vi "List Unacknowledged Packets.vi"(8 "error in (no error)":errorcluster, 9 "filter (0s: list all)":dbl, 11 "Subscription in":refnum<class "Subscription.lvclass">) -> (0 "error out":errorcluster, 2 "Unacknowledged":T1[](array[typedef]), 3 "Subscription out":refnum<class "Subscription.lvclass">)   [LabVIEW 2013, in "MQTT Server.lvlib" / "Subscription.lvclass"]
uses:
  Subscription.lvclass
  Stored Packet -- cluster.ctl
  <vilib>/LabVIEW Open Source Project/MQTT Control Packets/Control Packets/ControlPacket/ControlPacket.lvclass
  Subscription.lvclass/Subscription.ctl
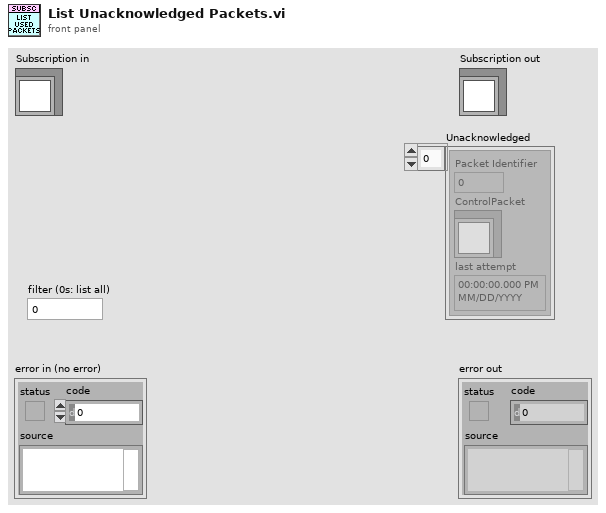
[diagram p1: front panel]
types:
  T1 = typedef "MQTT Server.lvlib/Subscription.lvclass/Stored Packet -- cluster.ctl" = cluster{"Packet Identifier":u16, "ControlPacket":refnum<class "ControlPacket.lvclass">, "last attempt":timestamp}
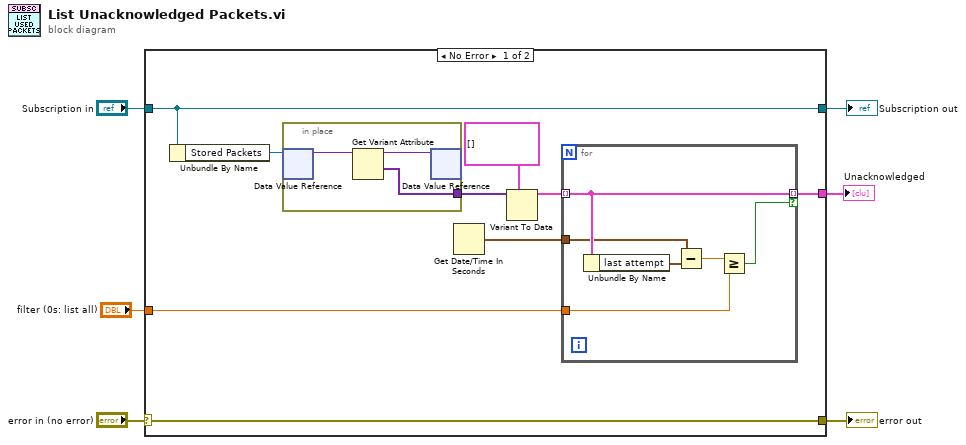
[diagram p0: block diagram]
diagram:
  n1 = case shown="No Error" "error in (no error)" {
    selector: "error in (no error)" -> [w15 w26]
    tunnel: [w15 w26] -> w5
    tunnel: [w14 w25] -> w3
    tunnel: "Subscription in" -> [w14 w25]
    tunnel: [w9 _] -> w2
    tunnel: "filter (0s: list all)" -> [w8 _]
    frame No Error {
      n2 = Unbundle By Name(w14) -> ("Stored Packets"=w13:refnum<data-value>)
      n3 = in-place {
        in-place-border: [w22] -> w12
        n4 = in-place-dvr #1(w13) -> (w24:variant)  [unwired: 1 out]
        n5 = Get Variant Attribute(Variant=w24) -> (duplicate Variant=w23:variant, values=w22:variant[])  [unwired: 3 in, 2 out]
        n6 = in-place-dvr #1(w23) -> ()  [unwired: 2 out]
      }
      n7 = Get Date/Time In Seconds() -> (seconds since 1Jan1904=w7:timestamp)
      n8 = Variant To Data(type=T1[] [], Variant=w12) -> (data=w10:T1[])  [unwired: 1 in, 1 out]
      n9 = for {
        tunnel: w10 -> [w21] mode=indexing
        tunnel: [w21] -> w9 mode=indexing if=w16
        tunnel: w8 -> [w17]
        tunnel: w7 -> [w20]
        n10 = Unbundle By Name(w21) -> ("last attempt"=w19:timestamp)
        n11 = Subtract(x=w20, y=w19) -> (x-y=w18:dbl)
        n12 = Greater Or Equal?(x=w18, y=w17) -> (x >= y?=w16:bool)
      }
    }
    frame Error {
    }
  }
  "error out" <- w5
  "Subscription out" <- w3
  "Unacknowledged" <- w2
